vi "Init.vi"() -> (14 "I/O":T24 {"IMU SPI A"."SPI Configuration"."Frame Length" min=1 max=16})   [LabVIEW 2018]
uses:
  <vilib>/myRIO/Instrument Drivers/Onboard IO/I2C/typedefs/I2C Reference.ctl
  <vilib>/myRIO/Common/Instrument Driver Framework/Utilities/typedefs/myRIO Generic Hardware Reference.ctl
  <vilib>/myRIO/Common/Instrument Driver Framework/Utilities/typedefs/Hardware Version Enum.ctl
  <vilib>/myRIO/Common/Instrument Driver Framework/Utilities/typedefs/myRIO v1.0 Reference.ctl
  <vilib>/myRIO/Common/Instrument Driver Framework/Utilities/typedefs/Generic FPGA Reference.ctl
  <vilib>/myRIO/Common/Instrument Driver Framework/myRIO v1.0/I2C/typedefs/I2C Channels Enum.ctl
  <vilib>/myRIO/Instrument Drivers/Onboard IO/I2C/typedefs/I2C Configuration.ctl
  <vilib>/myRIO/Instrument Drivers/Onboard IO/I2C/typedefs/I2C Transfer Rate.ctl
  <vilib>/myRIO/Instrument Drivers/Onboard IO/SPI/typedefs/SPI Reference.ctl
  <vilib>/myRIO/Common/Instrument Driver Framework/myRIO v1.0/SPI/typedefs/SPI Channels Enum.ctl
  <vilib>/myRIO/Instrument Drivers/Onboard IO/SPI/typedefs/SPI Configuration.ctl
  <vilib>/myRIO/Common/Instrument Driver Framework/myRIO v1.0/SPI/typedefs/SPI Clock Phase.ctl
  <vilib>/myRIO/Common/Instrument Driver Framework/myRIO v1.0/SPI/typedefs/SPI Clock Polarity.ctl
  <vilib>/myRIO/Common/Instrument Driver Framework/myRIO v1.0/SPI/typedefs/SPI Data Direction.ctl
  <vilib>/myRIO/Common/Instrument Driver Framework/myRIO v1.0/SPI/typedefs/SPI Frame Length.ctl
  <vilib>/myRIO/Instrument Drivers/Onboard IO/Encoder/typedefs/Encoder Reference.ctl
  <vilib>/myRIO/Common/Instrument Driver Framework/myRIO v1.0/Encoder/typedefs/Encoder Channels Enum.ctl
  <vilib>/myRIO/Instrument Drivers/Onboard IO/PWM/typedefs/PWM Reference.ctl
  <vilib>/myRIO/Common/Instrument Driver Framework/myRIO v1.0/PWM/typedefs/PWM Channels Enum.ctl
  <vilib>/myRIO/Instrument Drivers/Onboard IO/PWM/typedefs/PWM Configuration.ctl
  <vilib>/myRIO/Instrument Drivers/Onboard IO/DIO/typedefs/DIO Reference.ctl
  <vilib>/myRIO/Common/Instrument Driver Framework/myRIO v1.0/DIO/typedefs/DIO Channels List.ctl
  <vilib>/myRIO/Common/Instrument Driver Framework/myRIO v1.0/DIO/typedefs/DIO Channels Enum.ctl
  <vilib>/myRIO/Instrument Drivers/Onboard IO/I2C/typedefs/I2C User Configuration.ctl
  <vilib>/myRIO/Instrument Drivers/Onboard IO/SPI/typedefs/SPI User Configuration.ctl
  <vilib>/myRIO/Common/Instrument Driver Framework/myRIO v1.0/Encoder/typedefs/Encoder Signal Mode.ctl
  <vilib>/userdefined/High Color/nirio_resource_hc.ctl
  <vilib>/myRIO/Common/Instrument Driver Framework/myRIO v1.0/DIO/vis/myRIO v1.1 Open DIO.vi
  <vilib>/myRIO/Common/Instrument Driver Framework/myRIO v1.0/PWM/vis/myRIO v1.1 Open PWM.vi
  <vilib>/myRIO/Common/Instrument Driver Framework/Utilities/vis/Is FPGA Ref Available.vi
  <vilib>/myRIO/Common/Instrument Driver Framework/Utilities/vis/Validate Channels.vi
  <vilib>/myRIO/Common/Instrument Driver Framework/myRIO v1.0/DIO/vis/myRIO v1.0 Reserve DIO.vi
  <vilib>/myRIO/Common/Instrument Driver Framework/myRIO v1.0/PWM/vis/myRIO v1.0 Reserve PWM.vi
  <vilib>/myRIO/Common/Instrument Driver Framework/myRIO v1.0/Resource Manager/vis/myRIO v1.0 Reserve Channel List.vi
  <vilib>/myRIO/Common/Instrument Driver Framework/myRIO v1.0/DIO/vis/myRIO v1.0 Build MUX Configuration DIO.vi
  <vilib>/myRIO/Common/Instrument Driver Framework/myRIO v1.0/PWM/vis/myRIO v1.0 Build MUX Configuration PWM.vi
  <vilib>/myRIO/Common/Instrument Driver Framework/myRIO v1.0/Resource Manager/vis/myRIO v1.0 Reserve Channel.vi
  <vilib>/myRIO/Common/Instrument Driver Framework/myRIO v1.0/Resource Manager/vis/myRIO v1.0 Unreserve Channel.vi
  <vilib>/myRIO/Common/Instrument Driver Framework/myRIO v1.0/Resource Manager/vis/myRIO v1.0 Create Configuration List.vi
  <vilib>/myRIO/Common/Instrument Driver Framework/myRIO v1.0/Resource Manager/vis/myRIO v1.0 Build Mutex Name.vi
  <vilib>/Utility/error.llb/Error Cluster From Error Code.vi
  <vilib>/myRIO/Common/Instrument Driver Framework/myRIO v1.0/I2C/vis/myRIO v1.0 Configure I2C.vi
  <vilib>/myRIO/Common/Instrument Driver Framework/myRIO v1.0/SPI/vis/myRIO v1.0 Configure SPI.vi
  <vilib>/myRIO/Common/Instrument Driver Framework/myRIO v1.0/Encoder/vis/myRIO v1.0 Reset Encoder.vi
  <vilib>/Instr/_visa.llb/VISA Configure Serial Port (Instr).vi
  <vilib>/myRIO/Common/Instrument Driver Framework/myRIO v1.0/PWM/vis/myRIO v1.0 Write PWM.vi
  <vilib>/Utility/VariantDataType/GetNumericInfo.vi
  <vilib>/myRIO/Common/Instrument Driver Framework/myRIO v1.0/myRIO v1.1 Open.vi
  <vilib>/myRIO/Common/Instrument Driver Framework/Utilities/vis/IO Manager.vi
  <vilib>/myRIO/Common/Instrument Driver Framework/Utilities/vis/Configuration Manager.vi
  <vilib>/myRIO/Common/Instrument Driver Framework/myRIO v1.0/Resource Manager/vis/myRIO v1.0 Configure IO.vi
  <vilib>/myRIO/Common/Instrument Driver Framework/myRIO v1.0/myRIO v1.0 Close.vi
  <vilib>/myRIO/Common/Instrument Driver Framework/myRIO v1.0/DIO/vis/myRIO v1.0 Write DIO.vi
  <vilib>/myRIO/Express VI/Onboard IO/DO/DO Express VI.xnode
  <vilib>/myRIO/Instrument Drivers/Onboard IO/DIO/vis/myRIO DIO Open.xnode
  <vilib>/myRIO/Instrument Drivers/Onboard IO/PWM/vis/myRIO PWM Open.xnode
  <vilib>/myRIO/Instrument Drivers/Onboard IO/I2C/I2C.lvlib
  <vilib>/myRIO/Instrument Drivers/Onboard IO/DIO/DIO.lvlib
  <vilib>/myRIO/Instrument Drivers/Onboard IO/SPI/SPI.lvlib
  <vilib>/myRIO/Instrument Drivers/Onboard IO/Encoder/Encoder.lvlib
  <vilib>/myRIO/Instrument Drivers/Onboard IO/PWM/PWM.lvlib
panel:
  out "read buffer":string
  out "Lidar Mode":T17
  out "Lidar Pwr En":T17
  out "IMU SS":T17
  out "Tilt Servo PWM":T1
  out "Pan Servo PWM":T1
  out "GPS UART B":refnum<visa-resource-name>
  out "Left Encoder":T8
  out "Right Encoder":T8
  out "IMU SPI A":T10={"myRIO Reference"={"myRIO Model"=enum."Unknown", "myRIO Hardware Reference"={"Generic FPGA Reference"=refnum, "Allow multiple opens"=FALSE}}, "SPI Channels Enum"=enum."Not Connected", "SPI Configuration"={"Frequency [Hz]"=0.0, "Clock Phase"=enum."Leading", "Clock Polarity"=enum."Low", "Data Direction"=enum."Most significant bit first", "Frame Length"=8}} {"SPI Configuration"."Frame Length" min=1 max=16}
  out "Lidar I2C A":T20={"myRIO Reference"={"myRIO Model"=enum."Unknown", "myRIO Hardware Reference"={"Generic FPGA Reference"=refnum, "Allow multiple opens"=FALSE}}, "I2C Channels Enum"=enum."Not Connected", "I2C Configuration"={"I2C Transfer Rate"=enum."Fast mode (400 kbps)"}}
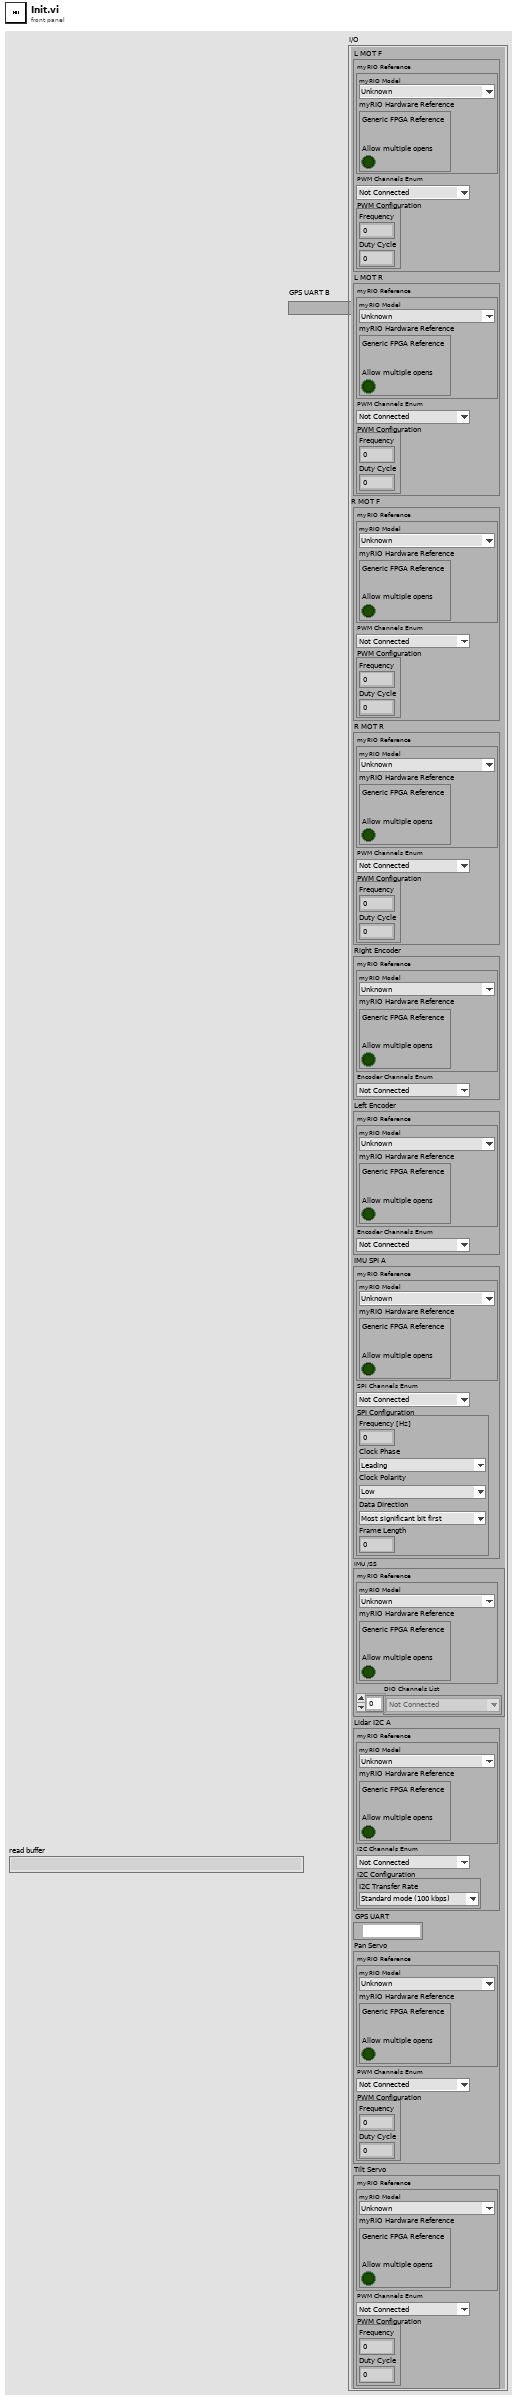
[diagram p1: front panel]
types:
  T1 = typedef "PWM.lvlib/PWM Reference.ctl" = cluster{"myRIO Reference":T2, "PWM Channels Enum":T6, "PWM Configuration":T7}
  T2 = typedef "myRIO Generic Hardware Reference.ctl" = cluster{"myRIO Model":T3, "myRIO Hardware Reference":T4}
  T3 = typedef "Hardware Version Enum.ctl" = enum16{"Unknown", "myRIO-1900", "myRIO-1950", "roboRIO", "NI ELVIS RIO CM", "ELVIS III"}
  T4 = typedef "myRIO v1.0 Reference.ctl" = cluster{"Generic FPGA Reference":T5, "Allow multiple opens":bool}
  T5 = typedef "Generic FPGA Reference.ctl" = refnum<k20>
  T6 = typedef "PWM Channels Enum.ctl" = enum16{"Not Connected", "C/PWM0", "C/PWM1", "A/PWM0", "A/PWM1", "A/PWM2", "A/PWM3", "A/PWM4", "A/PWM5", "A/PWM6", "A/PWM7", "A/PWM8", "A/PWM9", "A/PWM10", "A/PWM11", "A/PWM12", "A/PWM13", "A/PWM14", "A/PWM15", "A/PWM16", "A/PWM17", "A/PWM18", "A/PWM19", "B/PWM0", "B/PWM1", "B/PWM2", "B/PWM3", "B/PWM4", "B/PWM5", "B/PWM6", "B/PWM7", "B/PWM8", "B/PWM9", "B/PWM10", "B/PWM11", "B/PWM12", "B/PWM13", "B/PWM14", "B/PWM15", "B/PWM16", "B/PWM17", "B/PWM18", "B/PWM19", "PWM/PWM0", "PWM/PWM1", "PWM/PWM2", "PWM/PWM3", "PWM/PWM4", "PWM/PWM5", "PWM/PWM6", "PWM/PWM7", "PWM/PWM8", "PWM/PWM9"}
  T7 = typedef "PWM.lvlib/PWM Configuration.ctl" = cluster{"Frequency":dbl, "Duty Cycle":dbl}
  T8 = typedef "Encoder.lvlib/Encoder Reference.ctl" = cluster{"myRIO Reference":T2, "Encoder Channels Enum":T9}
  T9 = typedef "Encoder Channels Enum.ctl" = enum16{"Not Connected", "C/ENC0", "C/ENC1", "A/ENC", "A/ENC0", "A/ENC1", "A/ENC2", "A/ENC3", "A/ENC4", "A/ENC5", "A/ENC6", "A/ENC7", "A/ENC8", "A/ENC9", "B/ENC", "B/ENC0", "B/ENC1", "B/ENC2", "B/ENC3", "B/ENC4", "B/ENC5", "B/ENC6", "B/ENC7", "B/ENC8", "B/ENC9", "DIO/ENC0", "DIO/ENC1", "DIO/ENC2", "DIO/ENC3", "DIO/ENC4"}
  T10 = typedef "SPI.lvlib/SPI Reference.ctl" = cluster{"myRIO Reference":T2, "SPI Channels Enum":T11, "SPI Configuration":T12}
  T11 = typedef "SPI Channels Enum.ctl" = enum16{"Not Connected", "A/SPI", "B/SPI", "SPI/SPI"}
  T12 = typedef "SPI.lvlib/SPI Configuration.ctl" = cluster{"Frequency [Hz]":dbl, "Clock Phase":T13, "Clock Polarity":T14, "Data Direction":T15, "Frame Length":T16}
  T13 = typedef "SPI Clock Phase.ctl" = enum8{"Leading", "Trailing"}
  T14 = typedef "SPI Clock Polarity.ctl" = enum8{"Low", "High"}
  T15 = typedef "SPI Data Direction.ctl" = enum8{"Most significant bit first", "Least significant bit first"}
  T16 = typedef "SPI Frame Length.ctl" = u8
  T17 = typedef "DIO.lvlib/DIO Reference.ctl" = cluster{"myRIO Reference":T2, "DIO Channels List":T18}
  T18 = typedef "DIO Channels List.ctl" = T19[]
  T19 = typedef "DIO Channels Enum.ctl" = enum16{"Not Connected", "C/DIO0", "C/DIO1", "C/DIO2", "C/DIO3", "C/DIO4", "C/DIO5", "C/DIO6", "C/DIO7", "A/DIO0", "A/DIO1", "A/DIO2", "A/DIO3", "A/DIO4", "A/DIO5", "A/DIO6", "A/DIO7", "A/DIO8", "A/DIO9", "A/DIO10", "A/DIO11", "A/DIO12", "A/DIO13", "A/DIO14", "A/DIO15", "A/DIO16", "A/DIO17", "A/DIO18", "A/DIO19", "B/DIO0", "B/DIO1", "B/DIO2", "B/DIO3", "B/DIO4", "B/DIO5", "B/DIO6", "B/DIO7", "B/DIO8", "B/DIO9", "B/DIO10", "B/DIO11", "B/DIO12", "B/DIO13", "B/DIO14", "B/DIO15", "B/DIO16", "B/DIO17", "B/DIO18", "B/DIO19", "LED0", "LED1", "LED2", "LED3", "Button0", "DIO/DIO0", "DIO/DIO1", "DIO/DIO2", "DIO/DIO3", "DIO/DIO4", "DIO/DIO5", "DIO/DIO6", "DIO/DIO7", "DIO/DIO8", "DIO/DIO9", "SPI/CS0", "SPI/CS1", "SPI/CS2", "SPI/CS3", "LED RADIO (Green)", "LED RADIO (Red)", "LED COMM (Green)", "LED COMM (Red)", "LED MODE (Green)", "LED MODE (Red)"}
  T20 = typedef "I2C.lvlib/I2C Reference.ctl" = cluster{"myRIO Reference":T2, "I2C Channels Enum":T21, "I2C Configuration":T22}
  T21 = typedef "I2C Channels Enum.ctl" = enum16{"Not Connected", "A/I2C", "B/I2C", "I2C/I2C"}
  T22 = typedef "I2C.lvlib/I2C Configuration.ctl" = cluster{"I2C Transfer Rate":T23}
  T23 = typedef "I2C.lvlib/I2C Transfer Rate.ctl" = enum16{"Standard mode (100 kbps)", "Fast mode (400 kbps)"}
  T24 = cluster{"L MOT F":T1, "L MOT R":T1, "R MOT F":T1, "R MOT R":T1, "Right Encoder":T8, "Left Encoder":T8, "IMU SPI A":T10, "IMU /SS":T17, "Lidar I2C A":T20, "GPS UART":refnum<visa-resource-name>, "Pan Servo":T1, "Tilt Servo":T1}
  T25 = typedef "Encoder Signal Mode.ctl" = enum16{"Quadrature phase signal", "Step and direction signal"}
  T26 = typedef "SPI.lvlib/SPI User Configuration.ctl" = cluster{"Frequency [Hz]":dbl, "Clock Phase":T13, "Clock Polarity":T14, "Data Direction":T15, "Frame Length":T16}
  T27 = typedef "I2C.lvlib/I2C User Configuration.ctl" = cluster{"I2C Transfer Rate":T23}
  T28 = cluster{"PWM Ref Out":T1, "PWM Ref Out":T1, "PWM Ref Out":T1, "PWM Ref Out":T1, "Encoder Ref Out":T8, "Encoder Ref Out":T8, "SPI Ref Out":T10, "DIO Ref Out":T17, "I2C Ref Out":T20, "VISA resource name out":refnum<visa-resource-name>, "PWM Ref Out":T1, "PWM Ref Out":T1}
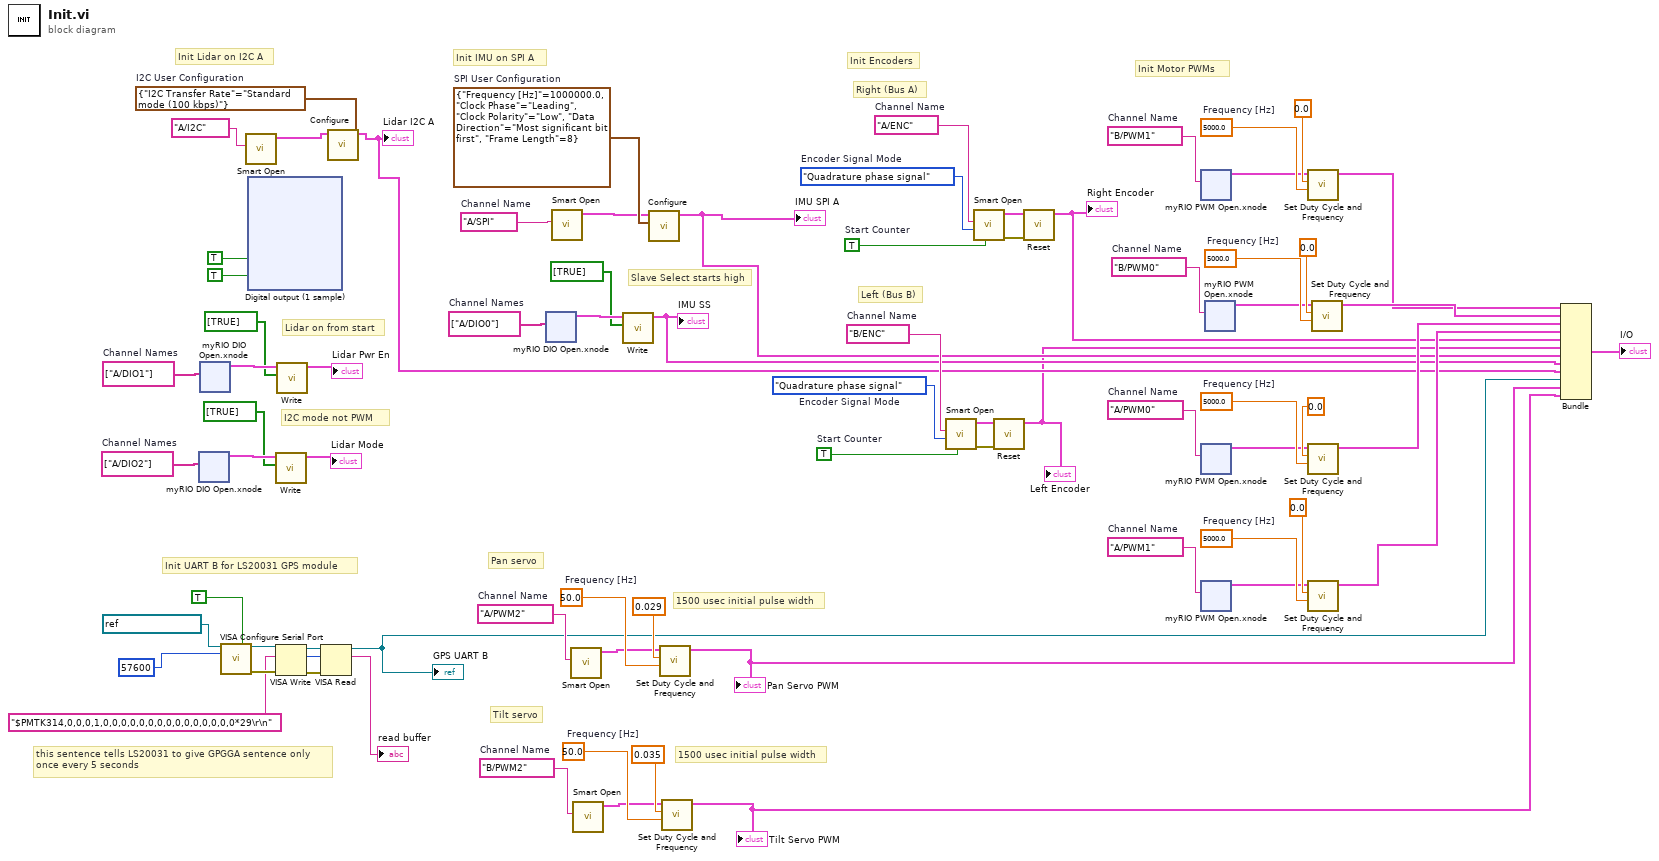
[diagram p0: block diagram]
diagram:
  w29 = tag[] ["A/DIO2"]  # Channel Names
  w33 = tag[] ["A/DIO1"]  # Channel Names
  w35 = 50.0  # Frequency [Hz]
  w37 = tag "B/PWM2"  # Channel Name
  w39 = 50.0  # Frequency [Hz]
  w41 = tag "A/PWM2"  # Channel Name
  w46 = 5000.0  # Frequency [Hz]
  w48 = tag "A/PWM1"  # Channel Name
  w50 = 5000.0  # Frequency [Hz]
  w52 = tag "A/PWM0"  # Channel Name
  w54 = 5000.0  # Frequency [Hz]
  w56 = tag "B/PWM0"  # Channel Name
  w57 = 5000.0  # Frequency [Hz]
  w59 = tag "B/PWM1"  # Channel Name
  w60 = TRUE  # Start Counter
  w61 = Encoder_Signal_Mode."Quadrature phase signal"  # Encoder Signal Mode
  w62 = tag "B/ENC"  # Channel Name
  w63 = TRUE  # Start Counter
  w64 = Encoder_Signal_Mode."Quadrature phase signal"  # Encoder Signal Mode
  w65 = tag "A/ENC"  # Channel Name
  w68 = tag[] ["A/DIO0"]  # Channel Names
  w70 = T26 {"Frequency [Hz]"=1000000.0, "Clock Phase"=enum."Leading", "Clock Polarity"=enum."Low", "Data Direction"=enum."Most significant bit first", "Frame Length"=8}  # SPI User Configuration
  w71 = tag "A/SPI"  # Channel Name
  w75 = T27 {"I2C Transfer Rate"=enum."Standard mode (100 kbps)"}  # I2C User Configuration
  # "this sentence tells LS20031 to give GPGGA sentence only\nonce every 5 seconds"
  # "I2C mode not PWM"
  # "Lidar on from start"
  # "Tilt servo"
  # "1500 usec initial pulse width"
  # "Pan servo"
  # "1500 usec initial pulse width"
  # "Init UART B for LS20031 GPS module"
  # "Init Motor PWMs"
  # "Left (Bus B)"
  # "Right (Bus A)"
  # "Init Encoders"
  # "Slave Select starts high"
  # "Init IMU on SPI A"
  # "Init Lidar on I2C A"
  n1 = xnode "myRIO DIO Open.xnode"("Channel Names"=w29) -> ("DIO Ref Out"=w28:T17)  [unwired: 2 in, 1 out]
  n2 = xnode "myRIO DIO Open.xnode"("Channel Names"=w33) -> ("DIO Ref Out"=w32:T17)  [unwired: 2 in, 1 out]
  n3 = call-poly "VISA Configure Serial Port"("VISA resource name"=refnum<visa-resource-name> "ASRL2::INSTR", "Enable Termination\nChar (T)"=TRUE ("Enable Termination\nChar (T)"), "baud rate (9600)"=u32 57600) -> ("VISA resource name out"=w7:refnum<visa-resource-name>, "error out"=w8:errorcluster)  [unwired: 11 in]
  n4 = call <vilib>:"Smart Open.vi"("Channel Name"=tag "A/I2C" ("I2C Channel Name")) -> ("I2C Ref Out"=w74:T20)  [unwired: 9 in, 1 out]
  n5 = xnode ("Digital output (1 sample)")("Lidar_pwr_en (A/DIO1 (Pin 13))"=TRUE, "Lidar_mode (A/DIO2 (Pin 15))"=TRUE) -> ()  [unwired: 1 in, 1 out]
  n6 = call <vilib>:"Write.vi"("Values"=bool[] [TRUE], "DIO Ref In"=w28) -> ("DIO Ref Out"=→"Lidar Mode":T17)  [unwired: 7 in, 1 out]
  n7 = VISA Write(VISA resource name=w7, write buffer="$PMTK314,0,0,0,1,0,0,0,0,0,0,0,0,0,0,0,0,0,0,0*29\r\n", error in (no error)=w8) -> (VISA resource name out=w3:refnum<visa-resource-name>, return count=w4:u32, error out=w5:errorcluster)
  n8 = call <vilib>:"Write.vi"("Values"=bool[] [TRUE], "DIO Ref In"=w32) -> ("DIO Ref Out"=→"Lidar Pwr En":T17)  [unwired: 7 in, 1 out]
  n9 = VISA Read(VISA resource name=w3, byte count=w4, error in (no error)=w5) -> (VISA resource name out=w2:refnum<visa-resource-name>, read buffer=→"read buffer":string)  [unwired: 2 out]
  "GPS UART B" <- w2
  n10 = call <vilib>:"Configure.vi"("I2C User Configuration"=w75, "I2C Ref In"=w74) -> ("I2C Ref Out"=w18:T20)  [unwired: 8 in, 1 out]
  "Lidar I2C A" <- w18
  n11 = xnode "myRIO DIO Open.xnode"("Channel Names"=w68) -> ("DIO Ref Out"=w67:T17)  [unwired: 2 in, 1 out]
  n12 = call <vilib>:"Smart Open.vi"("Channel Name"=w71) -> ("SPI Ref Out"=w69:T10)  [unwired: 9 in, 1 out]
  n13 = call <vilib>:"Smart Open.vi"("Channel Name"=w41) -> ("PWM Ref Out"=w38:T1)  [unwired: 9 in, 1 out]
  n14 = call <vilib>:"Smart Open.vi"("Channel Name"=w37) -> ("PWM Ref Out"=w34:T1)  [unwired: 9 in, 1 out]
  n15 = call <vilib>:"Write.vi"("Values"=bool[] [TRUE], "DIO Ref In"=w67) -> ("DIO Ref Out"=w19:T17)  [unwired: 7 in, 1 out]
  "IMU SS" <- w19
  n16 = call <vilib>:"Configure.vi"("SPI User Configuration"=w70, "SPI Ref In"=w69) -> ("SPI Ref Out"=w20:T10)  [unwired: 8 in, 1 out]
  "IMU SPI A" <- w20
  n17 = call <vilib>:"Set Duty Cycle and Frequency.vi"("Frequency [Hz]"=w39, "Duty Cycle"=0.029, "PWM Ref In"=w38) -> ("PWM Ref Out"=w17:T1)  [unwired: 6 in, 1 out]
  "Pan Servo PWM" <- w17
  n18 = call <vilib>:"Set Duty Cycle and Frequency.vi"("Frequency [Hz]"=w35, "Duty Cycle"=0.035, "PWM Ref In"=w34) -> ("PWM Ref Out"=w16:T1)  [unwired: 6 in, 1 out]
  "Tilt Servo PWM" <- w16
  n19 = call <vilib>:"Smart Open.vi"("Start Counter"=w60, "Encoder Signal Mode"=w61, "Channel Name"=w62) -> ("error out"=w11:errorcluster, "Encoder Ref Out"=w10:T8)  [unwired: 7 in]
  n20 = call <vilib>:"Smart Open.vi"("Start Counter"=w63, "Encoder Signal Mode"=w64, "Channel Name"=w65) -> ("error out"=w14:errorcluster, "Encoder Ref Out"=w13:T8)  [unwired: 7 in]
  n21 = call <vilib>:"Reset.vi"("error in (no error)"=w11, "Encoder Ref In"=w10) -> ("Encoder Ref Out"=w9:T8)  [unwired: 8 in, 1 out]
  "Left Encoder" <- w9
  n22 = call <vilib>:"Reset.vi"("error in (no error)"=w14, "Encoder Ref In"=w13) -> ("Encoder Ref Out"=w12:T8)  [unwired: 8 in, 1 out]
  "Right Encoder" <- w12
  n23 = xnode "myRIO PWM Open.xnode"("Channel Name"=w59) -> ("PWM Ref Out"=w25:T1)  [unwired: 2 in, 1 out]
  n24 = xnode "myRIO PWM Open.xnode"("Channel Name"=w52) -> ("PWM Ref Out"=w49:T1)  [unwired: 2 in, 1 out]
  n25 = xnode "myRIO PWM Open.xnode"("Channel Name"=w48) -> ("PWM Ref Out"=w45:T1)  [unwired: 2 in, 1 out]
  n26 = xnode "myRIO PWM Open.xnode"("Channel Name"=w56) -> ("PWM Ref Out"=w53:T1)  [unwired: 2 in, 1 out]
  n27 = call <vilib>:"Set Duty Cycle and Frequency.vi"("Frequency [Hz]"=w57, "Duty Cycle"=0.0, "PWM Ref In"=w25) -> ("PWM Ref Out"=w21:T1)  [unwired: 6 in, 1 out]
  n28 = call <vilib>:"Set Duty Cycle and Frequency.vi"("Frequency [Hz]"=w50, "Duty Cycle"=0.0, "PWM Ref In"=w49) -> ("PWM Ref Out"=w23:T1)  [unwired: 6 in, 1 out]
  n29 = call <vilib>:"Set Duty Cycle and Frequency.vi"("Frequency [Hz]"=w46, "Duty Cycle"=0.0, "PWM Ref In"=w45) -> ("PWM Ref Out"=w22:T1)  [unwired: 6 in, 1 out]
  n30 = call <vilib>:"Set Duty Cycle and Frequency.vi"("Frequency [Hz]"=w54, "Duty Cycle"=0.0, "PWM Ref In"=w53) -> ("PWM Ref Out"=w24:T1)  [unwired: 6 in, 1 out]
  n31 = Bundle("PWM Ref Out"=w21, "PWM Ref Out"=w24, "PWM Ref Out"=w23, "PWM Ref Out"=w22, "Encoder Ref Out"=w12, "Encoder Ref Out"=w9, "SPI Ref Out"=w20, "DIO Ref Out"=w19, "I2C Ref Out"=w18, "VISA resource name out"=w2, "PWM Ref Out"=w17, "PWM Ref Out"=w16) -> (→"I/O":T28)  [unwired: 1 in]
